vi "Read from Stream.vi"(10 "Stream in":refnum<class "Stream.lvclass">, 11 "LabVIEW Binary in":refnum<class "LabVIEW Binary.lvclass">) -> (0 "error out":errorcluster, 2 "Message Data":T1)   [LabVIEW 2020, in "Stream-Simple-Msg.lvlib" / "LabVIEW Binary.lvclass"]
uses:
  LabVIEW Binary.lvclass
  <vilib>/IlluminatedG/lv-stream/stream/Stream.lvclass
  Message/Message Data.ctl
  Message/Message___.lvclass
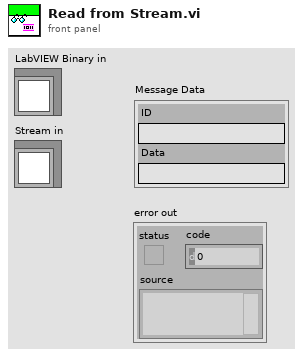
[diagram p1: front panel]
types:
  T1 = typedef "Stream-Simple-Msg.lvlib/Message___.lvclass/Message Data.ctl" = cluster{"ID":string, "Data":string}
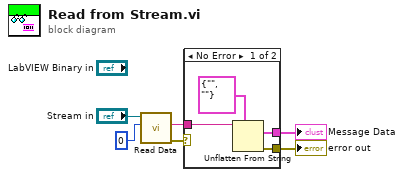
[diagram p0: block diagram]
diagram:
  n1 = call <vilib>:"Read Data.vi"("Count"=0, "Stream in"="Stream in") -> ("error out"=w1:errorcluster, "Data"=w3:string)  [unwired: 7 in, 1 out]
  n2 = case shown="No Error" w1 {
    selector: w1 -> [_ w11]
    tunnel: [w9 _] -> w5
    tunnel: [w8 w11] -> w4
    tunnel: w3 -> [w7 _]
    frame No Error {
      n3 = Unflatten From String(type=T1 {"ID"="", "Data"=""} ("Message Data"), binary string=w7) -> (value=w9:T1, error out=w8:errorcluster)  [unwired: 3 in, 1 out]
    }
    frame Error {
    }
  }
  "error out" <- w4
  "Message Data" <- w5
